vi "Simplex_Engine.vi"(0 "Simplex Parameters":dbl[](array[numeric]), 2 "Actions":T1=enum."Compute Centroid", 7 "x Values - Amount of Modes":dbl[][](array[numeric])) -> (8 "Test X":dbl[](array[numeric]))   [LabVIEW 2014]
doc: "Compute the Simplex reflection, expansion, contraction and reduction assuming the worst point (f of x) has been sorted into the first array element. That is, we ignore the first column of the input.\n\nSimplex Parameters assumes the values are in the following order:\n\nAlpha - Reflection coefficient\nBeta - Expansion coefficient\nGamma - Contraction coefficient\nOther - Reduction coefficient (Not Used)"
uses:
  Simplex_Engine_Controls.ctl
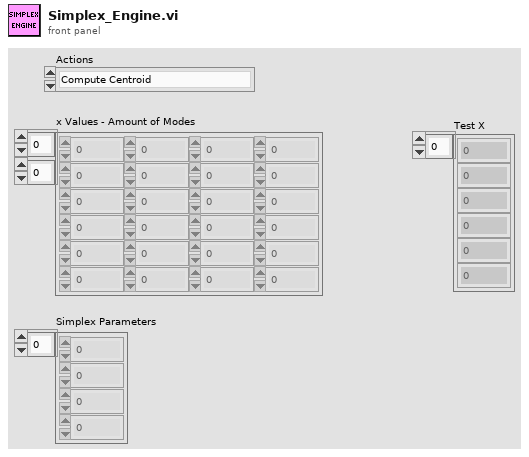
[diagram p1: front panel]
types:
  T1 = typedef "Simplex_Engine_Controls.ctl" = enum16{"Initialize", "Compute Centroid", "Sort", "Evaluate", "Switch", "Get Reflection", "Get Expansion", "Get Contraction", "Get Reduction", "Exit"}
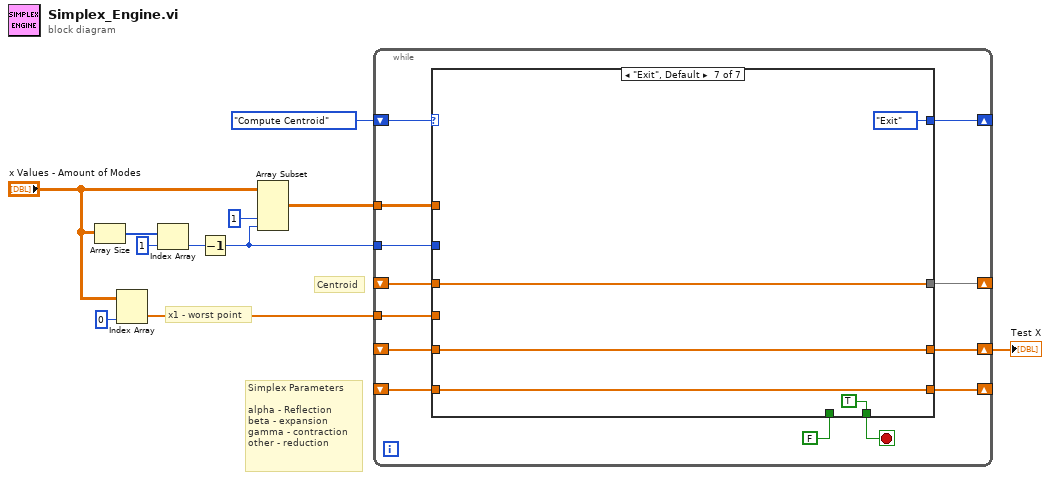
[diagram p0: block diagram]
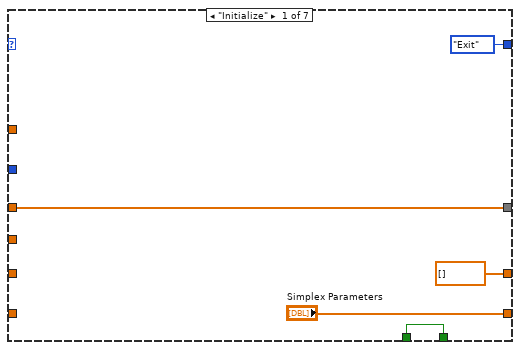
[diagram p2: hidden frame]
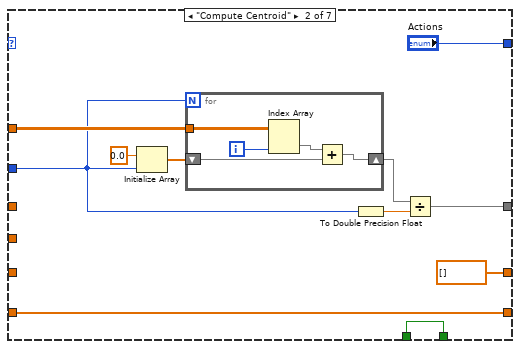
[diagram p3: hidden frame]
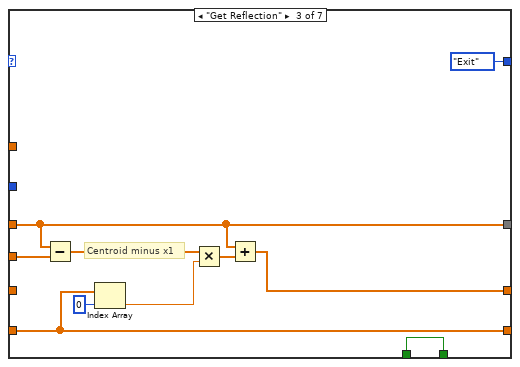
[diagram p4: hidden frame]
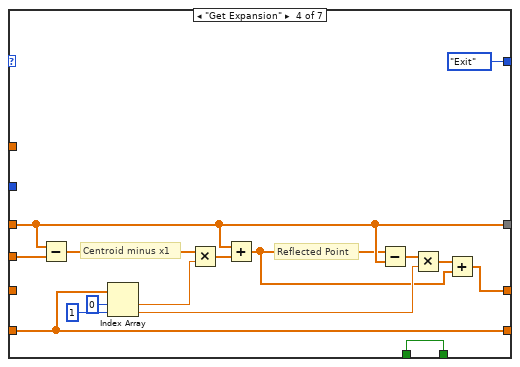
[diagram p5: hidden frame]
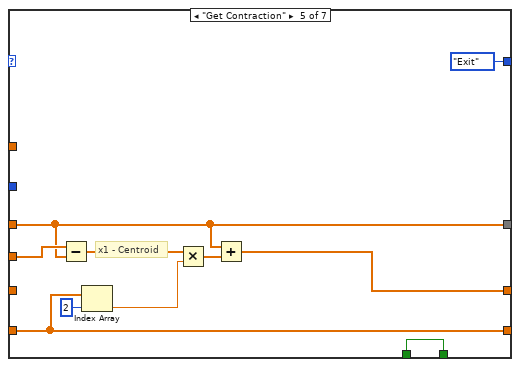
[diagram p6: hidden frame]
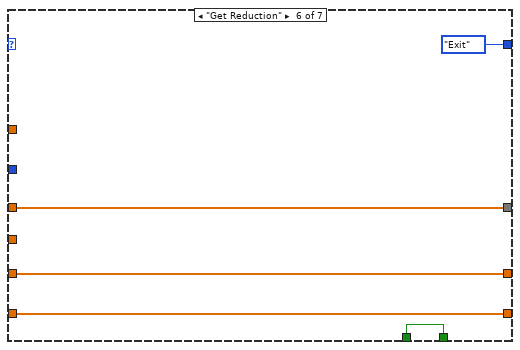
[diagram p7: hidden frame]
diagram:
  # "x1 - worst point"
  # "Simplex Parameters\n\nalpha - Reflection\nbeta - expansion\ngamma - contraction\nother - reduction"
  # "Centroid"
  n1 = Array Size(array="x Values - Amount of Modes") -> (size(s)=w10:i32[])
  n2 = Index Array(array="x Values - Amount of Modes", index (col)=0 ("disabled index (col)")) -> (element=w2:dbl[])  [unwired: 1 in]
  n3 = Index Array(array=w10, index=1) -> (element=w8:i32)
  n4 = Decrement(x=w8) -> (x-1=w6:i32)
  n5 = Array Subset(array="x Values - Amount of Modes", index (col)=1 ("index"), length (col)=w6) -> (w7:dbl[][])  [unwired: 2 in]
  n6 = while {
    tunnel: w7 -> [w24]
    tunnel: w6 -> [w23]
    shift-right: [w22] -> _
    shift-left: Simplex_Engine_Controls."Compute Centroid" ("Actions") -> [w21]
    shift-right: [w20] -> _
    shift-left: _ -> [w19]
    shift-right: [w18] -> _
    shift-left: _ -> [w17]
    tunnel: w2 -> [w16]
    shift-right: [w13] -> w1
    shift-left: _ -> [w12]
    stop <- w14 stop-if-true
    n7 = case shown="\"Exit\", Default" w21 {
      tunnel: w24 -> [_ w38 _ _ _ _ _]
      tunnel: w23 -> [_ w36 _ _ _ _ _]
      tunnel: [Simplex_Engine_Controls."Exit" ("Actions") "Actions" Simplex_Engine_Controls."Exit" ("Actions") Simplex_Engine_Controls."Exit" ("Actions") Simplex_Engine_Controls."Exit" ("Actions") Simplex_Engine_Controls."Exit" ("Actions") Simplex_Engine_Controls."Exit" ("Actions")] -> w22
      tunnel: [w29 w33 w49 w61 w74 w85 w86] -> w20
      tunnel: w19 -> [w29 _ w49 w61 w74 w85 w86]
      tunnel: ["Simplex Parameters" w32 w53 w64 w78 w82 w88] -> w18
      tunnel: w17 -> [_ w32 w53 w64 w78 w82 w88]
      tunnel: w16 -> [_ _ w55 w65 w80 _ _]
      tunnel: FALSE -> [w26 w31 w48 w62 w73 w83 _]
      tunnel: [w26 w31 w48 w62 w73 w83 TRUE] -> w14
      tunnel: [dbl[] [] dbl[] [] w47 w56 w72 w81 w87] -> w13
      tunnel: w12 -> [_ _ _ _ _ w81 w87]
      frame "Initialize" {
      }
      frame "Compute Centroid" {
        n8 = Initialize Array(0.0 ("element"), w36) -> (w39:dbl[])
        n9 = for {
          N: w36 -> [_]
          shift-right: [w44] -> w37
          shift-left: w39 -> [w45]
          tunnel: w38 -> [w43]
          i -> [w41]
          n10 = Index Array(array=w43, index (col)=w41) -> (element=w42:dbl[])  [unwired: 1 in]
          n11 = Add(x=w42, y=w45) -> (x+y=w44:dbl[])
        }
        n12 = To Double Precision Float(number=w36) -> (double precision float=w35:dbl)
        n13 = Divide(x=w37, y=w35) -> (x/y=w33:dbl[])
      }
      frame "Get Reflection" {
        # "Centroid minus x1"
        n14 = Subtract(x=w49, y=w55) -> (x-y=w54:dbl[])
        n15 = Index Array(array=w53, index=0) -> (element=w51:dbl)
        n16 = Multiply(x=w54, y=w51) -> (x*y=w50:dbl[])
        n17 = Add(x=w49, y=w50) -> (x+y=w47:dbl[])
      }
      frame "Get Expansion" {
        # "Reflected Point"
        # "Centroid minus x1"
        n18 = Subtract(x=w61, y=w65) -> (x-y=w66:dbl[])
        n19 = Index Array(array=w64, index #1=0 ("index"), index #2=1 ("index")) -> (element #1=w68:dbl, element #2=w59:dbl)
        n20 = Multiply(x=w66, y=w68) -> (x*y=w69:dbl[])
        n21 = Add(x=w61, y=w69) -> (x+y=w57:dbl[])
        n22 = Subtract(x=w57, y=w61) -> (x-y=w60:dbl[])
        n23 = Multiply(x=w60, y=w59) -> (x*y=w58:dbl[])
        n24 = Add(x=w58, y=w57) -> (x+y=w56:dbl[])
      }
      frame "Get Contraction" {
        # "x1 - Centroid"
        n25 = Subtract(x=w80, y=w74) -> (x-y=w79:dbl[])
        n26 = Index Array(array=w78, index=2) -> (element=w76:dbl)
        n27 = Multiply(x=w79, y=w76) -> (x*y=w75:dbl[])
        n28 = Add(x=w74, y=w75) -> (x+y=w72:dbl[])
      }
      frame "Get Reduction" {
      }
      frame "Exit", Default {
      }
    }
  }
  "Test X" <- w1
